vi "-8781 Channel Identifier not found--error.vi"(8 "error in":errorcluster, 11 "Channel Identifier":string) -> (0 "error out":errorcluster)   [LabVIEW 2024, in "Thermometer Multichannel Worker.lvlib" / "Thermometer Multichannel Worker.lvclass"]
uses:
  Thermometer Multichannel Worker.lvclass
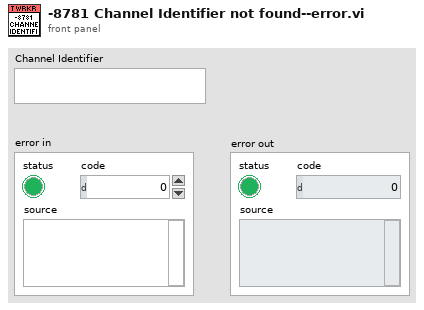
[diagram p1: front panel]
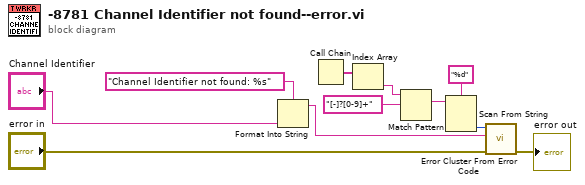
[diagram p0: block diagram]
diagram:
  n1 = Format Into String(format string="Channel Identifier not found: %s" ("error message (\"\")"), "Channel Identifier") -> (resulting string=w2:string)  [unwired: 2 in, 1 out]
  n2 = Call Chain() -> (call chain=w9:string[])
  n3 = Index Array(array=w9) -> (element=w7:string)  [unwired: 1 in]
  n4 = Match Pattern(string=w7, regular expression="[-]?[0-9]+") -> (match substring=w6:string)  [unwired: 1 in, 3 out]
  n5 = Scan From String(format string="%d", input string=w6) -> (output 1=w4:i32)  [unwired: 3 in, 3 out]
  n6 = call <vilib>:"Error Cluster From Error Code.vi"("error in (no error)"="error in", "error message (\"\")"=w2, "error code (0)"=w4) -> ("error out"=→"error out":errorcluster)  [unwired: 6 in]
